vi "Detect Packet Size Error.vi"(7 "reset_pse":bool, 8 "end of frame":bool, 9 "input valid":bool, 10 "packet_header":bool, 11 "chdr_header":T3) -> (1 "eof_misalignment_count":u64, 2 "sequence errors":T2, 3 "packet size errors":T1)   [LabVIEW 2023, in "CHDR Support.lvlib"]
doc: "Checks for dropped packets and packet size errors by counting valid inputs and comparing to the expected values provided by the header. Includes testing that the header follows an end of frame signal and that the next header's sequence number is 1 greater than the previous."
uses:
  CHDR Support.lvlib
  <instrlib>/_niInstr/Basic Elements/v1/FPGA/niInstr Basic Elements v1 FPGA.lvlib
  <instrlib>/_niInstr/Basic Elements/v1/FPGA/Private/Count Up U64.vi
  CHDR Header Layout.ctl
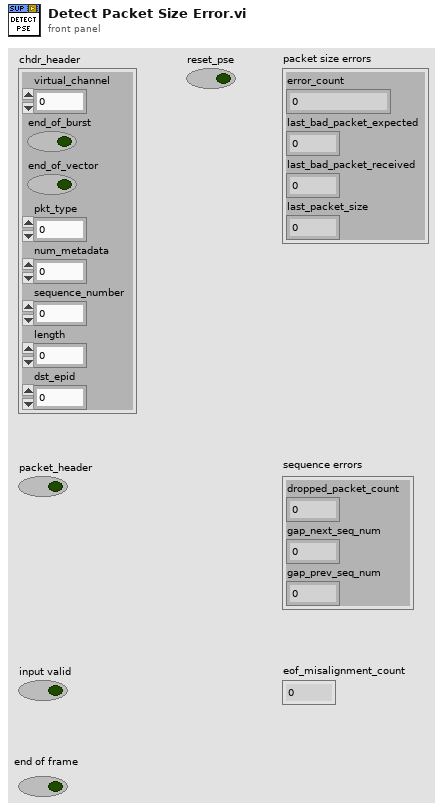
[diagram p1: front panel]
types:
  T1 = cluster{"error_count":u64, "last_bad_packet_expected":u16, "last_bad_packet_received":u16, "last_packet_size":u16}
  T2 = cluster{"dropped_packet_count":u64, "gap_next_seq_num":u16, "gap_prev_seq_num":u16}
  T3 = typedef "CHDR Support.lvlib/CHDR Header Layout.ctl" = cluster{"virtual_channel":fxp<+,6,6>, "end_of_burst":bool, "end_of_vector":bool, "pkt_type":fxp<+,3,3>, "num_metadata":fxp<+,5,5>, "sequence_number":u16, "length":u16, "dst_epid":u16}
  T4 = cluster{u64, "sequence_number":u16, "sequence_number":u16}
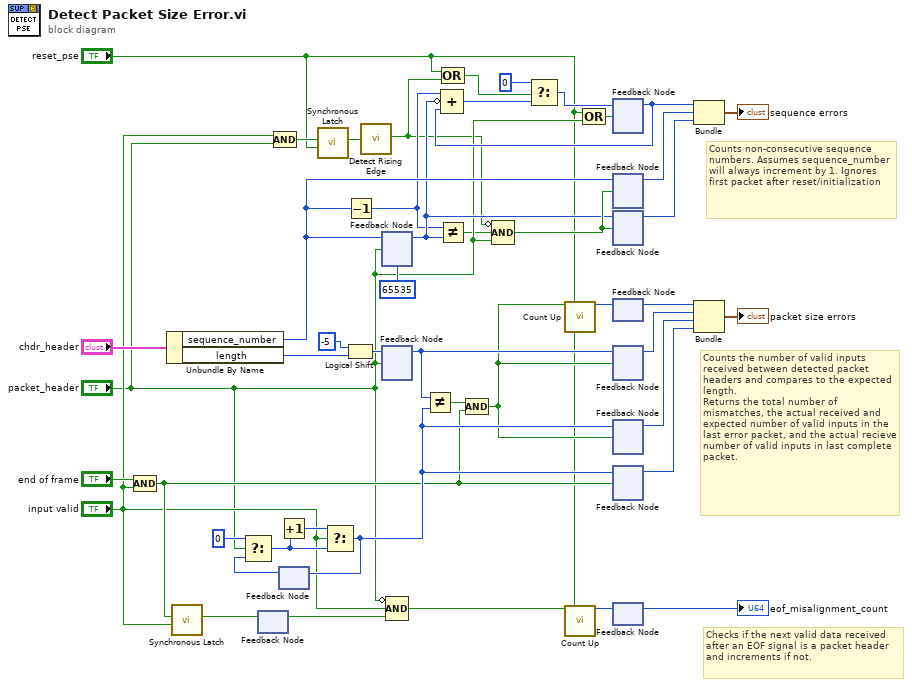
[diagram p0: block diagram]
diagram:
  # "Checks if the next valid data received after an EOF signal is a packet header and increments if not."
  # "Counts the number of valid inputs received between detected packet headers and compares to the expected length.\nReturns the total number of mismatches, the actual received and expected number of valid inputs in the last error packet, and the actual recieve number of valid inputs in last complete packet."
  # "Counts non-consecutive sequence numbers. Assumes sequence_number will always increment by 1. Ignores first packet after reset/initialization"
  n1 = Compound Arithmetic op=AND("end of frame", "input valid") -> (w20:bool)
  n2 = Unbundle By Name("chdr_header") -> ("sequence_number"=w31:u16, "length"=w45:u16)
  n3 = call <instrlib>:"Synchronous Latch.vi"("clear"="input valid", "set"=w20) -> ("out"=w32:bool)  [unwired: 9 in]
  n4 = feedback #1() -> (w21:bool)  [unwired: 1 in]
  n5 = feedback-in #1(w32) -> ()
  n6 = Compound Arithmetic op=AND("input valid", "packet_header") -> (w6:bool)
  n7 = feedback #2() -> (w36:u16)  [unwired: 1 in]
  n8 = Select(t=u16 0, s="packet_header", f=w36) -> (s? t:f=w38:u16)
  n9 = Increment(x=w38) -> (x+1=w39:u16)
  n10 = call <instrlib>:"Synchronous Latch.vi"("clear"="reset_pse", "set"=w6) -> ("out"=w3:bool)  [unwired: 9 in]
  n11 = Select(t=w39, s="input valid", f=w38) -> (s? t:f=w35:u16)
  n12 = feedback-in #2(w35) -> ()
  n13 = Logical Shift(y=i16 -5, x=w45) -> (x << y=w42:u16)
  n14 = Decrement(x=w31) -> (x-1=w29:u16)
  n15 = call <instrlib>:"Detect Rising Edge.vi"("signal"=w3) -> ("edge detected"=w1:bool)  [unwired: 14 in]
  n16 = feedback #3(u16 65535 ("sequence_number")) -> (w30:u16)
  n17 = feedback-in #3(w31, "packet_header") -> ()
  n18 = feedback #4() -> (w41:u16)  [unwired: 1 in]
  n19 = feedback-in #4(w42, "packet_header") -> ()
  n20 = Compound Arithmetic op=AND(invert "packet_header", "input valid", w21) -> (w24:bool)
  n21 = Not Equal?(x=w41, y=w35) -> (x != y?=w40:bool)
  n22 = Not Equal?(x=w29, y=w30) -> (x != y?=w2:bool)
  n23 = Compound Arithmetic op=OR("reset_pse", w1) -> (w4:bool)
  n24 = Compound Arithmetic op=AND(w40, w20) -> (w19:bool)
  n25 = Compound Arithmetic op=AND(invert w1, w2, "packet_header") -> (w34:bool)
  n26 = call-poly <instrlib>:"Count Up.vi"("increment"=w19, "reset"="reset_pse") -> ("count out"=w43:u64)  [unwired: 13 in]
  n27 = call-poly <instrlib>:"Count Up.vi"("increment"=w24, "reset"="reset_pse") -> ("count out"=w23:u64)  [unwired: 13 in]
  n28 = Compound Arithmetic op=OR("reset_pse", "packet_header") -> (w25:bool)
  n29 = feedback #5() -> (w18:u64)  [unwired: 1 in]
  n30 = Compound Arithmetic op=ADD(w29, invert w30, w18) -> (w27:u64)
  n31 = Select(t=u64 0, s=w4, f=w27) -> (s? t:f=w26:u64)
  n32 = feedback-in #5(w26, w25) -> ()
  n33 = feedback #6() -> (w17:u16)  [unwired: 1 in]
  n34 = feedback-in #6(w31, w34) -> ()
  n35 = feedback #7() -> (w16:u16)  [unwired: 1 in]
  n36 = feedback-in #7(w30, w34) -> ()
  n37 = feedback #8() -> (w14:u64)  [unwired: 1 in]
  n38 = feedback-in #8(w43) -> ()
  n39 = feedback #9() -> (w13:u16)  [unwired: 1 in]
  n40 = feedback-in #9(w41, w19) -> ()
  n41 = feedback #10() -> (w12:u16)  [unwired: 1 in]
  n42 = feedback-in #10(w35, w19) -> ()
  n43 = feedback #11() -> (w11:u16)  [unwired: 1 in]
  n44 = feedback-in #11(w35, w20) -> ()
  n45 = feedback #12() -> (→"eof_misalignment_count":u64)  [unwired: 1 in]
  n46 = feedback-in #12(w23) -> ()
  n47 = Bundle(w18, "sequence_number"=w17, "sequence_number"=w16) -> (→"sequence errors":T4)  [unwired: 1 in]
  n48 = Bundle("count out"=w14, w13, w12, w11) -> (→"packet size errors":cluster{"count out":u64, u16, u16, u16})  [unwired: 1 in]
